vi "Load RSL File.vi"(8 "error in (no error)":errorcluster, 11 "RSL Path":path) -> (0 "error out":errorcluster, 2 "invalid file?":bool, 3 "RSL Data":T9 {"Test Config Data"."Test Ranking" items=["Low", "Normal", "High"]})   [LabVIEW 2019]
uses:
  <vilib>/addons/analyzer/_analyzerctrls.llb/VIAnCtl Results.ctl
  <vilib>/addons/analyzer/_analyzerctrls.llb/VIAnCtl ResultsData (index).ctl
  <vilib>/addons/analyzer/_analyzerctrls.llb/VIAnCtl ResultStatus.ctl
  <vilib>/addons/analyzer/_vianresshared.llb/VIAnRes Parsed Results Data (by VI).ctl
  <vilib>/addons/analyzer/_vianresshared.llb/VIAnRes Parsed Results Data (by Test).ctl
  <vilib>/addons/analyzer/_analyzerctrls.llb/VIAnCtl Test Config Data.ctl
  <vilib>/addons/analyzer/_analyzerctrls.llb/VIAnCtl TestRanking.ctl
  <vilib>/addons/analyzer/_analyzerctrls.llb/VIAnCtl Config Control Value.ctl
panel:
  in  "old rsl":string="This RSL file was saved with LabVIEW 2017 or previous. Object highlighting in the VI Analyzer Results Window is not supported with older RSL files in LabVIEW 2018 and later."
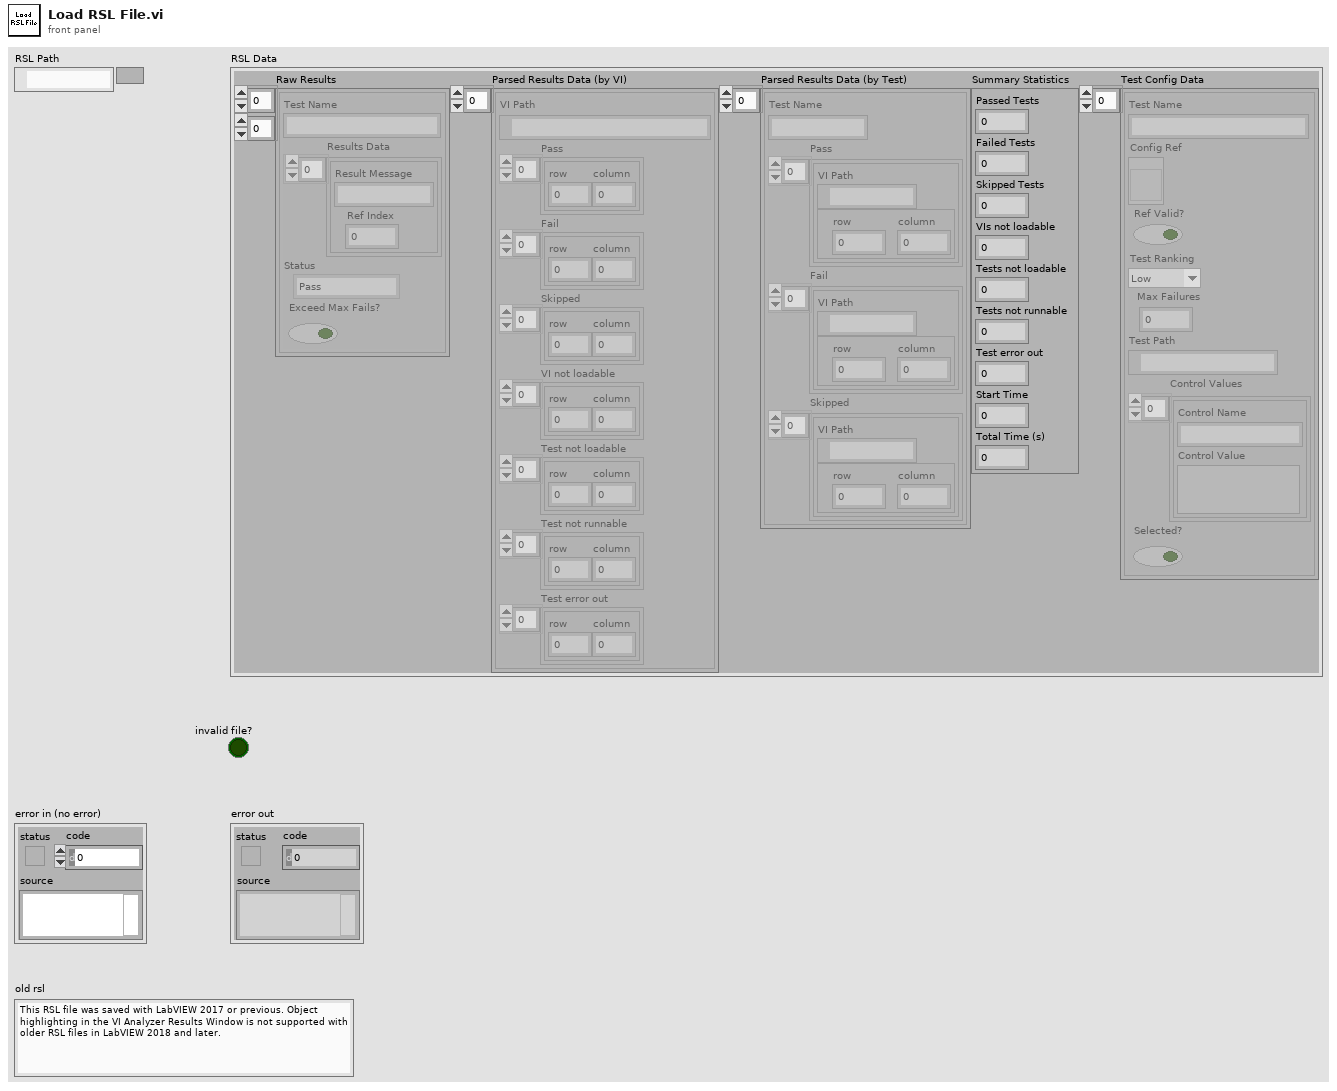
[diagram p1: front panel]
types:
  T1 = typedef "VIAnCtl Results.ctl" = cluster{"Test Name":string, "Results Data":T2[], "Status":T3, "Exceed Max Fails?":bool}
  T2 = typedef "VIAnCtl ResultsData (index).ctl" = cluster{"Result Message":string, "Ref Index":i32}
  T3 = typedef "VIAnCtl ResultStatus.ctl" = enum16{"Pass", "Fail", "Skipped", "VI not loadable", "Test not loadable", "Test not runnable", "Test error out"}
  T4 = typedef "VIAnRes Parsed Results Data (by VI).ctl" = cluster{"VI Path":path, "Pass":cluster{"row":i32, "column":i32}[], "Fail":cluster{"row":i32, "column":i32}[], "Skipped":cluster{"row":i32, "column":i32}[], "VI not loadable":cluster{"row":i32, "column":i32}[], "Test not loadable":cluster{"row":i32, "column":i32}[], "Test not runnable":cluster{"row":i32, "column":i32}[], "Test error out":cluster{"row":i32, "column":i32}[]}
  T5 = typedef "VIAnRes Parsed Results Data (by Test).ctl" = cluster{"Test Name":string, "Pass":cluster{"VI Path":path, "index":cluster{"row":i32, "column":i32}}[], "Fail":cluster{"VI Path":path, "index":cluster{"row":i32, "column":i32}}[], "Skipped":cluster{"VI Path":path, "index":cluster{"row":i32, "column":i32}}[]}
  T6 = typedef "VIAnCtl Test Config Data.ctl" = cluster{"Test Name":string, "Config Ref":refnum<vi>, "Ref Valid?":bool, "Test Ranking":T7, "Max Failures":u32, "Test Path":path, "Control Values":T8[], "Selected?":bool}
  T7 = typedef "VIAnCtl TestRanking.ctl" = u16
  T8 = typedef "VIAnCtl Config Control Value.ctl" = cluster{"Control Name":string, "Control Value":variant}
  T9 = cluster{"Raw Results":T1[][], "Parsed Results Data (by VI)":T4[], "Parsed Results Data (by Test)":T5[], "Summary Statistics":cluster{"Passed Tests":i32, "Failed Tests":i32, "Skipped Tests":i32, "VIs not loadable":i32, "Tests not loadable":i32, "Tests not runnable":i32, "Test error out":i32, "Start Time":u32, "Total Time (s)":dbl}, "Test Config Data":T6[]}
  T10 = cluster{"Passed Tests":i32, "Failed Tests":i32, "Skipped Tests":i32, "VIs not loadable":i32, "Tests not loadable":i32, "Tests not runnable":i32, "Test error out":i32, "Start Time":u32, "Total Time (s)":dbl}
  T11 = cluster{"Pass":i32, "Fail":i32, "Skipped":i32, "VI not loadable":i32, "Test not loadable":i32, "Test not runnable":i32, "Test error out":i32}
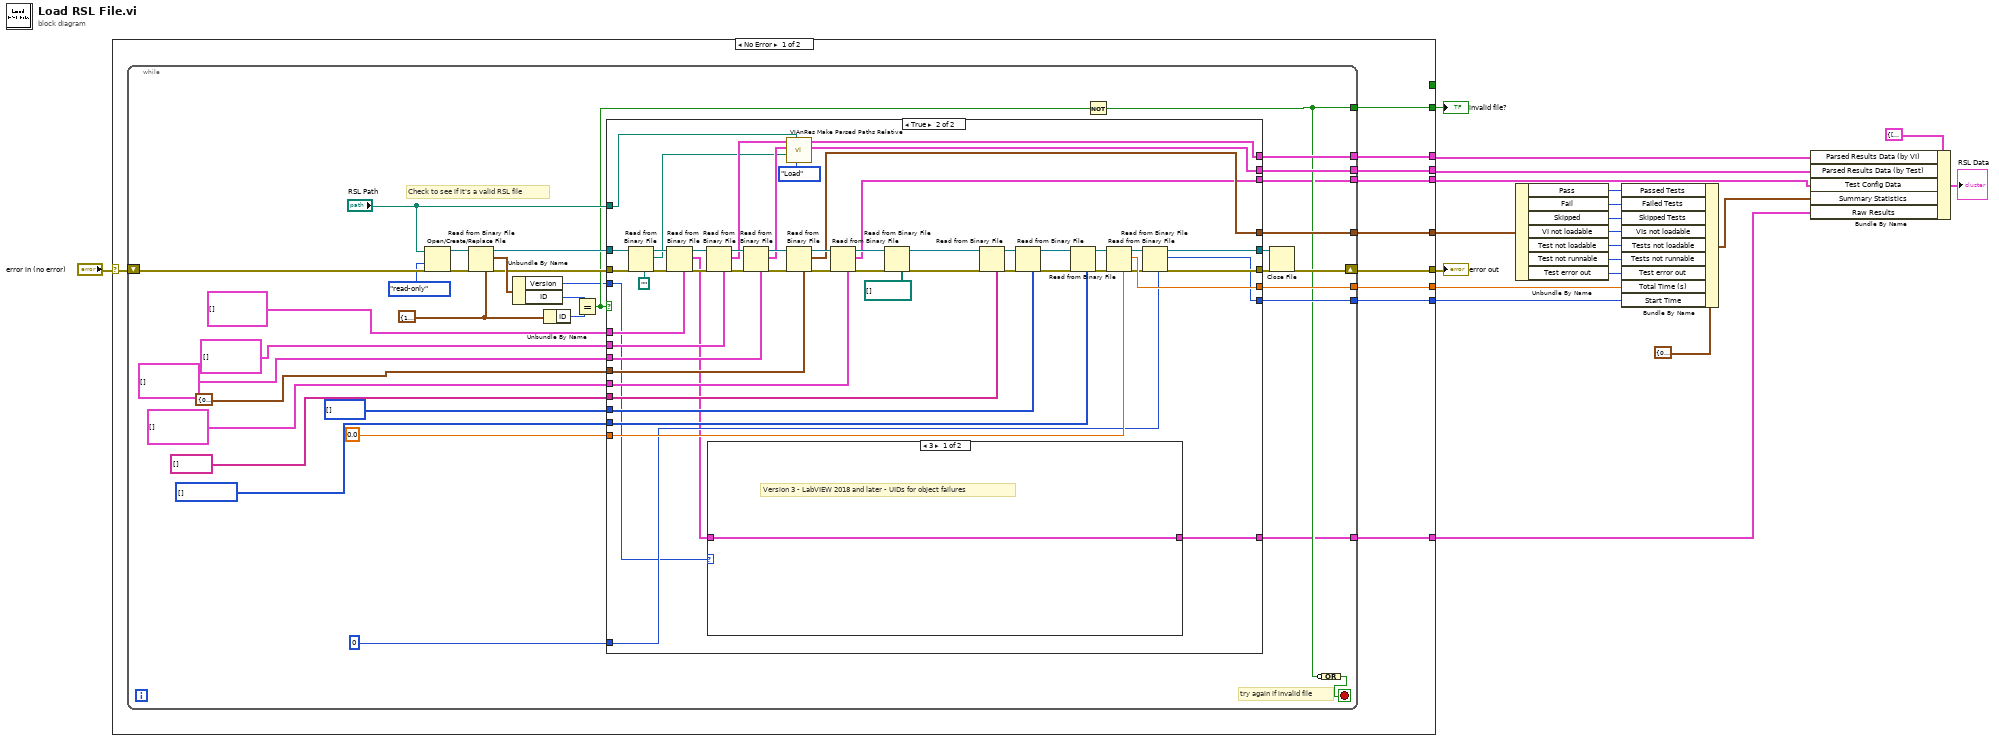
[diagram p0: block diagram]
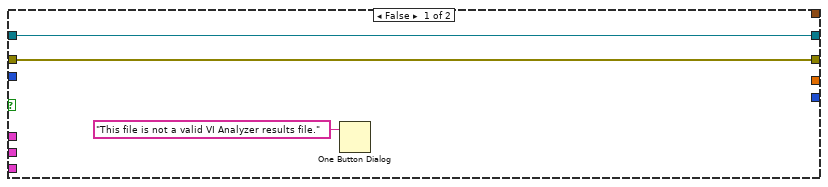
[diagram p2: hidden frame]
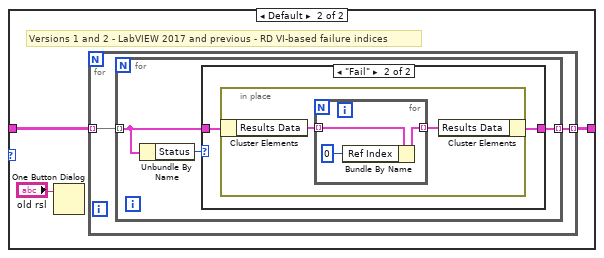
[diagram p3: hidden frame]
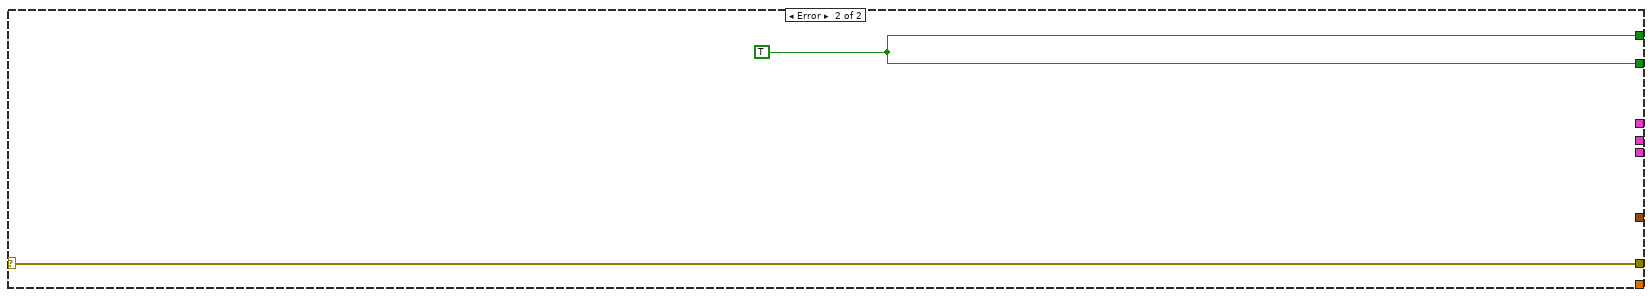
[diagram p5: hidden frame]
diagram:
  n1 = case shown="No Error" "error in (no error)" {
    selector: "error in (no error)" -> [w24 w140]
    tunnel: [w31 w140] -> w20
    tunnel: [_ w139] -> _
    tunnel: [w30 w139] -> w19
    tunnel: [w29 _] -> w17
    tunnel: [w28 _] -> w16
    tunnel: [w27 _] -> w14
    tunnel: [w26 _] -> w5
    tunnel: [w25 _] -> w6
    tunnel: [w23 _] -> w4
    tunnel: [w22 _] -> w2
    frame No Error {
      n2 = while {
        tunnel: [w48] -> w30
        tunnel: [w58] -> w29
        tunnel: [w57] -> w28
        tunnel: [w56] -> w27
        tunnel: [w54] -> w26
        tunnel: [w53] -> w25
        shift-right: [w66] -> w31
        shift-left: w24 -> [w50]
        tunnel: [w34] -> w23
        tunnel: [w33] -> w22
        stop <- w49 stop-if-true
        w32 = cluster{"ID":i32, "Version":i32} {"ID"=1934326086, "Version"=3} ("File Info")
        w59 = T7[] [] items=["Low", "Normal", "High"] ("dum Rankings")
        # "Check to see if it's a valid RSL file"
        # "try again if invalid file"
        n3 = Open/Create/Replace File(file path (use dialog)="RSL Path", error in=w50, access (0:read/write)=enum16{"read/write", "read-only", "write-only"}."read-only") -> (refnum out=w36:refnum<file>, error out=w37:errorcluster)  [unwired: 4 out]
        n4 = Read from Binary File ("Read File")(5:w32, 8:w37, 11:w36) -> (0:w43:errorcluster, 2:w46:cluster{"ID":i32, "Version":i32}, 3:w42:refnum<file>)  [unwired: 4 out]
        n5 = Unbundle By Name(w46) -> ("Version"=w35:i32, "ID"=w45:i32)
        n6 = Unbundle By Name(w32) -> ("ID"=w44:i32)
        n7 = Equal?(x=w45, y=w44) -> (x = y?=w41:bool)
        n8 = case shown="True" w41 {
          tunnel: w43 -> [w68 w80]
          tunnel: w42 -> [w69 w79]
          tunnel: [w68 w100] -> w39
          tunnel: T4[] [] ("dum Parsed Results Data (by VI)") -> [_ w121]
          tunnel: T5[] [] ("dum Parsed Results Data (by Test)") -> [_ w120]
          tunnel: T11 {"Pass"=0, "Fail"=0, "Skipped"=0, "VI not loadable"=0, "Test not loadable"=0, "Test not runnable"=0, "Test error out"=0} ("dum Numbers") -> [_ w117]
          tunnel: T6[] [] ("dum Test Config Data") -> [_ w114]
          tunnel: u32[] [] ("dum Max Failures") -> [_ w113]
          tunnel: [w69 w99] -> w40
          tunnel: string[] [] ("dum Tags") -> [_ w110]
          tunnel: w59 -> [_ w105]
          tunnel: [_ w83] -> w58
          tunnel: [_ w82] -> w57
          tunnel: [_ w86] -> w56
          tunnel: 0.0 ("dum Tot Time") -> [_ w102]
          tunnel: [_ w101] -> w54
          tunnel: [_ w96] -> w53
          tunnel: u32 0 ("dum Timestamp") -> [_ w95]
          tunnel: "RSL Path" -> [_ w74]
          tunnel: T1[][] [] ("dum Raw Data") -> [_ w92]
          tunnel: w35 -> [_ w73]
          tunnel: [_ w71] -> w34
          tunnel: [_ w70] -> w33
          frame False {
            n9 = One Button Dialog(message="This file is not a valid VI Analyzer results file.") -> ()  [unwired: 2 out]
          }
          frame True {
            n10 = Read from Binary File ("Read File")(5:path "", 8:w80, 11:w79) -> (0:w77:errorcluster, 2:w75:path, 3:w78:refnum<file>)  [unwired: 4 out]
            n11 = Read from Binary File ("Read File")(5:w92, 8:w77, 11:w78) -> (0:w93:errorcluster, 2:w72:T1[][], 3:w94:refnum<file>)  [unwired: 4 out]
            n12 = Read from Binary File ("Read File")(5:w121, 8:w93, 11:w94) -> (0:w108:errorcluster, 2:w85:T4[], 3:w109:refnum<file>)  [unwired: 4 out]
            n13 = case shown="3" w73 {
              tunnel: [w122 w124] -> w71
              tunnel: w72 -> [w122 w125]
              frame 3 {
                # "Version 3 - LabVIEW 2018 and later - UIDs for object failures"
              }
              frame Default {
                # "Versions 1 and 2 - LabVIEW 2017 and previous - RD VI-based failure indices"
                n14 = One Button Dialog(message="old rsl") -> ()  [unwired: 1 in, 1 out]
                n15 = for {
                  tunnel: w125 -> [w127] mode=indexing
                  tunnel: [w126] -> w124 mode=indexing
                  n16 = for {
                    tunnel: w127 -> [w129] mode=indexing
                    tunnel: [w128] -> w126 mode=indexing
                    n17 = Unbundle By Name(w129) -> ("Status"=w130:T3)
                    n18 = case shown="\"Fail\"" w130 {
                      tunnel: w129 -> [w131 w133]
                      tunnel: [w131 w132] -> w128
                      frame Default {
                      }
                      frame "Fail" {
                        n19 = in-place {
                          n20 = in-place-cluster #1(w133) -> ("Results Data"=w135:T2[])
                          n21 = for {
                            tunnel: w135 -> [w138] mode=indexing
                            tunnel: [w137] -> w134 mode=indexing
                            n22 = Bundle By Name(cluster=w138, "Ref Index"=0) -> (w137:T2)
                          }
                          n23 = in-place-cluster #1("Results Data"=w134) -> (w132:T1)
                        }
                      }
                    }
                  }
                }
              }
            }
            n24 = Read from Binary File ("Read File")(5:w120, 8:w108, 11:w109) -> (0:w118:errorcluster, 2:w84:T5[], 3:w119:refnum<file>)  [unwired: 4 out]
            n25 = call <vilib>:"VIAnRes Make Parsed Paths Relative.vi"("Op"=enum16{"Load", "Save"}."Load", "Current RSL Path"=w74, "Stored RSL Path"=w75, "Parsed Results Data (by Test) in"=w84, "Parsed Results Data (by VI) in"=w85) -> ("Parsed Results Data (by Test) out"=w82:T5[], "Parsed Results Data (by VI) out"=w83:T4[])  [unwired: 5 out]
            n26 = Read from Binary File ("Read File")(5:w117, 8:w118, 11:w119) -> (0:w115:errorcluster, 2:w86:T11, 3:w116:refnum<file>)  [unwired: 4 out]
            n27 = Read from Binary File ("Read File")(5:w114, 8:w115, 11:w116) -> (0:w90:errorcluster, 2:w70:T6[], 3:w91:refnum<file>)  [unwired: 4 out]
            n28 = Read from Binary File ("Read File")(5:path[] [], 8:w90, 11:w91) -> (0:w88:errorcluster, 3:w89:refnum<file>)  [unwired: 5 out]
            n29 = Read from Binary File ("Read File")(5:w110, 8:w88, 11:w89) -> (0:w111:errorcluster, 3:w112:refnum<file>)  [unwired: 5 out]
            n30 = Read from Binary File ("Read File")(5:w113, 8:w111, 11:w112) -> (0:w106:errorcluster, 3:w107:refnum<file>)  [unwired: 5 out]
            n31 = Read from Binary File ("Read File")(5:w105, 8:w106, 11:w107) -> (0:w103:errorcluster, 3:w104:refnum<file>)  [unwired: 5 out]
            n32 = Read from Binary File ("Read File")(5:w102, 8:w103, 11:w104) -> (0:w97:errorcluster, 2:w101:dbl, 3:w98:refnum<file>)  [unwired: 4 out]
            n33 = Read from Binary File ("Read File")(5:w95, 8:w97, 11:w98) -> (0:w100:errorcluster, 2:w96:u32, 3:w99:refnum<file>)  [unwired: 4 out]
          }
        }
        n34 = Not(x=w41) -> (.not. x?=w48:bool)
        n35 = Close File(refnum=w40, error in=w39) -> (error out=w66:errorcluster)  [unwired: 1 out]
        n36 = Compound Arithmetic op=OR(invert w48) -> (w49:bool)
      }
    }
    frame Error {
      w139 = TRUE
    }
  }
  "error out" <- w20
  "invalid file?" <- w19
  n37 = Unbundle By Name(w14) -> ("Pass"=w7:i32, "Fail"=w8:i32, "Skipped"=w9:i32, "VI not loadable"=w10:i32, "Test not loadable"=w13:i32, "Test not runnable"=w12:i32, "Test error out"=w11:i32)
  n38 = Bundle By Name(cluster=T10 {"Passed Tests"=0, "Failed Tests"=0, "Skipped Tests"=0, "VIs not loadable"=0, "Tests not loadable"=0, "Tests not runnable"=0, "Test error out"=0, "Start Time"=0, "Total Time (s)"=0.0} ("Summary Statistics"), "Passed Tests"=w7, "Failed Tests"=w8, "Skipped Tests"=w9, "VIs not loadable"=w10, "Tests not loadable"=w13, "Tests not runnable"=w12, "Test error out"=w11, "Total Time (s)"=w5, "Start Time"=w6) -> (w3:T10)
  n39 = Bundle By Name(cluster=T9 {"Raw Results"=[], "Parsed Results Data (by VI)"=[], "Parsed Results Data (by Test)"=[], "Summary Statistics"={"Passed Tests"=0, "Failed Tests"=0, "Skipped Tests"=0, "VIs not loadable"=0, "Tests not loadable"=0, "Tests not runnable"=0, "Test error out"=0, "Start Time"=0, "Total Time (s)"=0.0}, "Test Config Data"=[]} ("Analysis Results"), "Parsed Results Data (by VI)"=w17, "Parsed Results Data (by Test)"=w16, "Test Config Data"=w2, "Summary Statistics"=w3, "Raw Results"=w4) -> (→"RSL Data":T9)
